vi "Global communication.vi"() -> ()   [LabVIEW 2016]
panel:
  in  "Status":dbl[](array[numeric])
  in  "RPF":dbl[](array[numeric])
  in  "Reserved15":dbl[](array[numeric])
  in  "Reserved14":dbl[](array[numeric])
  in  "Reserved13":dbl[](array[numeric])
  in  "MAG-C-R":dbl[](array[numeric])
  in  "MAG-C-L":dbl[](array[numeric])
  in  "MAG-B-R":dbl[](array[numeric])
  in  "MAG-B-L":dbl[](array[numeric])
  in  "MAG-A-R":dbl[](array[numeric])
  in  "MAG-A-L":dbl[](array[numeric])
  in  "FREQ-R":dbl[](array[numeric])
  in  "FREQ-L":dbl[](array[numeric])
  in  "APF":dbl[](array[numeric])
  in  "ANG-DIFF":dbl[](array[numeric])
  in  "Global communication":dbl[](array[numeric])
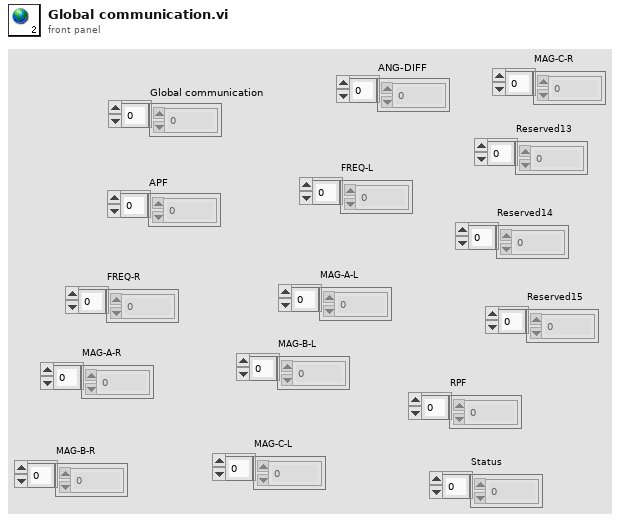
[diagram p1: front panel]
diagram:
